vi "XNET Example IP Stack Config - Multiple VLANs.vi"(0 "XNET interface":refnum<k21>, 5 "VLANs":T1[](array[typedef]), 11 "error in (no error)":errorcluster) -> (4 "config":string, 15 "error out":errorcluster)   [LabVIEW 2018]
doc: "This example subVI generates a JSON configuration string for use with XNET IP Stack Create.vi. The configuration string supports a single XNET interface (physical interface) and one or more VLANs (virtual interfaces), each with a static IPv4 address, and a static IPv6 address.\nYou can re-use this subVI in one of two ways: a) copy the subVI from the example diagram to your VI diagram, which re-uses the subVI unchanged (located in the XNET library), or b) use Save As to create a copy of the subVI in your application folder, and change as needed."
uses:
  XNET Example IP Stack Config - Simple VLAN.ctl
  XNET Example IP Stack Config - Stack.ctl
  XNET Example IP Stack Config - XNET Interface.ctl
  XNET Example IP Stack Config - MAC.ctl
  XNET Example IP Stack Config - VLAN.ctl
  XNET Example IP Stack Config - Static Address.ctl
  XNET Example IP Stack Config - Static IPv6 Address.ctl
  XNET Example IP Stack Config - Proxy Server.ctl
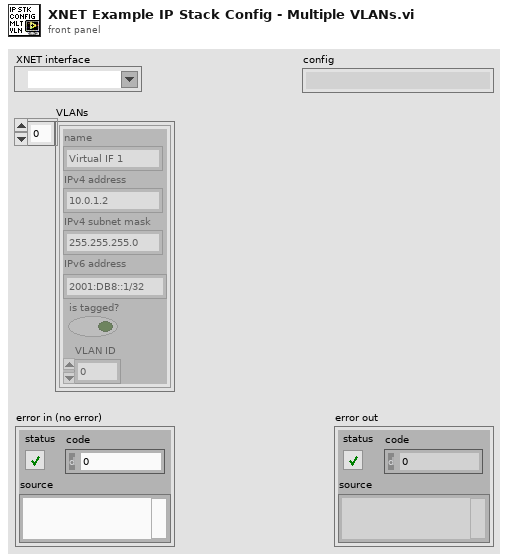
[diagram p1: front panel]
types:
  T1 = typedef "XNET Example IP Stack Config - Simple VLAN.ctl" = cluster{"name":string, "IPv4 address":string, "IPv4 subnet mask":string, "IPv6 address":string, "is tagged?":bool, "VLAN ID":u16}
  T2 = typedef "XNET Example IP Stack Config - MAC.ctl" = cluster{"address":string, "VLANs":T3[]}
  T3 = typedef "XNET Example IP Stack Config - VLAN.ctl" = cluster{"name":string, "isTagged":bool, "id":u16, "IPv4":cluster{"mode":string, "staticAddresses":T4[]}, "IPv6":cluster{"mode":string, "staticAddresses":T5[]}}
  T4 = typedef "XNET Example IP Stack Config - Static Address.ctl" = cluster{"address":string, "subnetMask":string}
  T5 = typedef "XNET Example IP Stack Config - Static IPv6 Address.ctl" = cluster{"address":string}
  T6 = typedef "XNET Example IP Stack Config - XNET Interface.ctl" = cluster{"name":string, "MACs":T2[]}
  T7 = typedef "XNET Example IP Stack Config - Stack.ctl" = cluster{"schema":string, "xnetInterfaces":T6[], "proxyServers":T8[]}
  T8 = typedef "XNET Example IP Stack Config - Proxy Server.ctl" = cluster{"protocol":string, "direction":string, "listenAddress":string, "listenPort":u16, "forwardingDestinationAddress":string, "forwardingDestinationPort":u16, "forwardingSourceAddress":string, "forwardingSourcePort":u16}
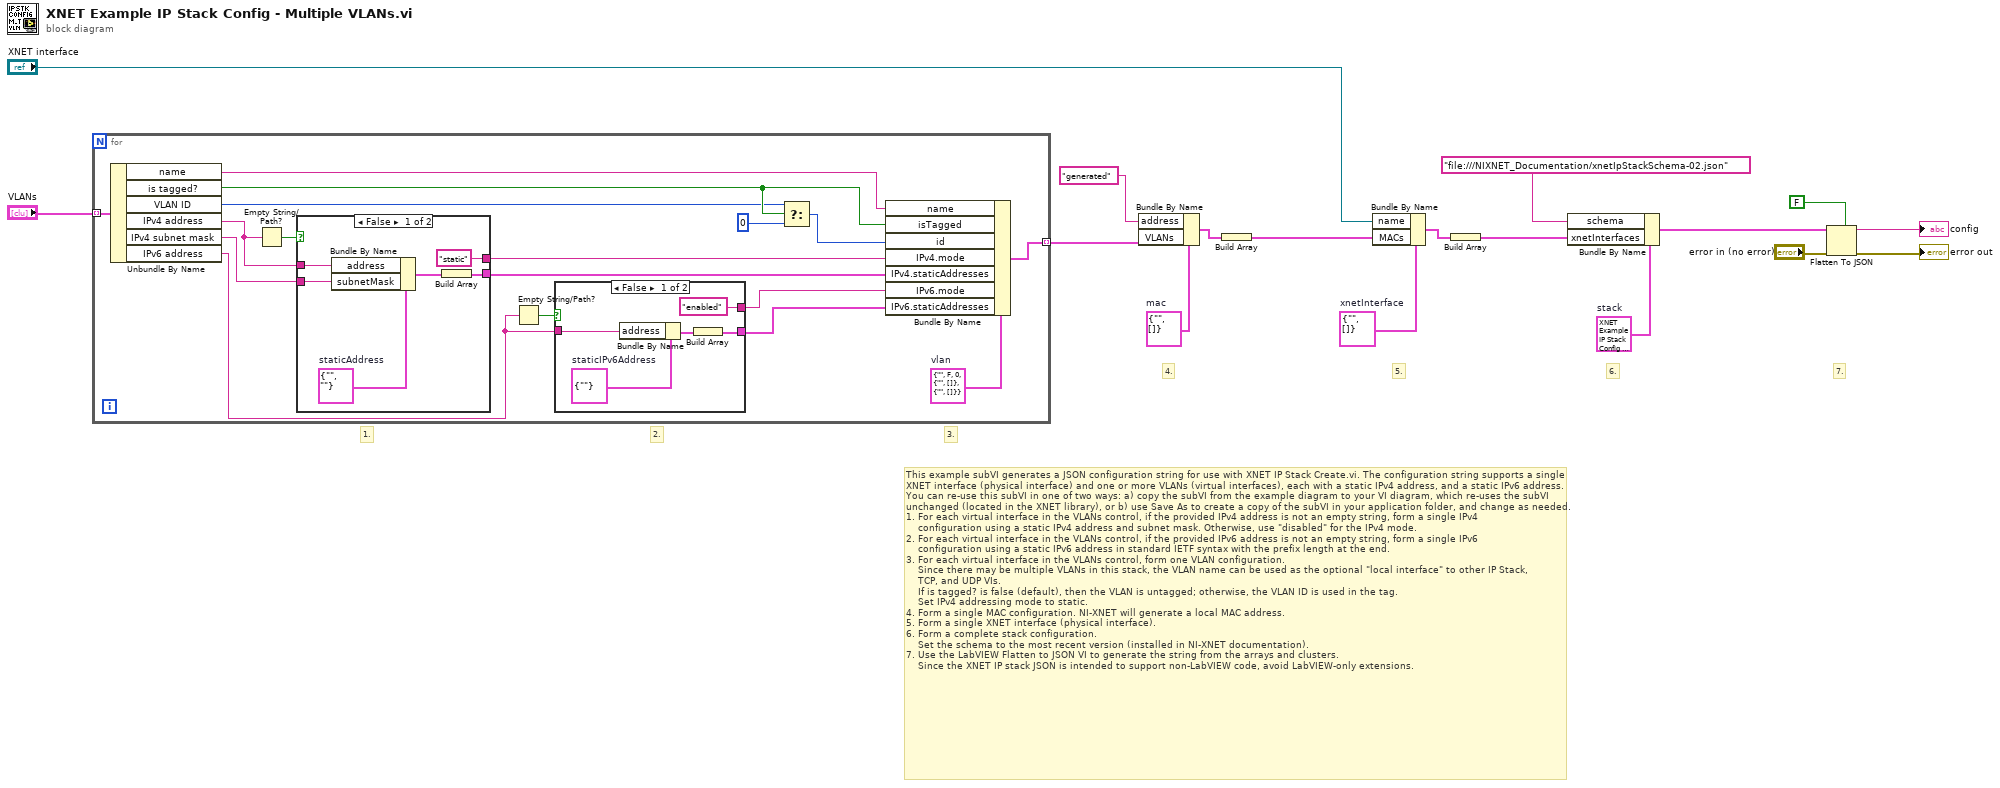
[diagram p0: block diagram]
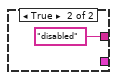
[diagram p2: hidden frame]
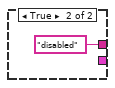
[diagram p3: hidden frame]
diagram:
  w6 = T2 {"address"="", "VLANs"=[]}  # mac
  w9 = T6 {"name"="", "MACs"=[]}  # xnetInterface
  w10 = T7 {"schema"="", "xnetInterfaces"=[{"name"="", "MACs"=[{"address"="", "VLANs"=[{"name"="", "isTagged"=FALSE, "id"=0, "IPv4"={"mode"="static", "staticAddresses"=[]}, "IPv6"={"mode"="", "staticAddresses"=[]}}]}]}], "proxyServers"=[]}  # stack
  # "2."
  # "1."
  # "3."
  # "7."
  # "6."
  # "5."
  # "4."
  # "This example subVI generates a JSON configuration string for use with XNET IP Stack Create.vi. The configuration string supports a single XNET interface (physical interface) and one or more VLANs (virtual interfaces), each with a static IPv4 address, and a static IPv6 address.\nYou can re-use this subVI in one of two ways: a) copy the subVI from the example diagram to your VI diagram, which re-uses the subVI unchanged (located in the XNET library), or b) use Save As to create a copy of the subVI in your application folder, and change as needed.\n1. For each virtual interface in the VLANs control, if the provided IPv4 address is not an empty string, form a single IPv4\n    configuration using a static IPv4 address and subnet mask. Otherwise, use \"disabled\" for the IPv4 mode.\n2. For each virtual interface in the VLANs control, if the provided IPv6 address is not an empty string, form a single IPv6\n    configuration using a static IPv6 address in standard IETF syntax with the prefix length at the end.\n3. For each virtual interface in the VLANs control, form one VLAN configuration.\n    Since there may be multiple VLANs in this stack, the VLAN name can be used as the optional \"local interface\" to other IP Stack,     \n    TCP, and UDP VIs.\n    If is tagged? is false (default), then the VLAN is untagged; otherwise, the VLAN ID is used in the tag.\n    Set IPv4 addressing mode to static.\n4. Form a single MAC configuration. NI-XNET will generate a local MAC address.\n5. Form a single XNET interface (physical interface).\n6. Form a complete stack configuration.\n    Set the schema to the most recent version (installed in NI-XNET documentation).\n7. Use the LabVIEW Flatten to JSON VI to generate the string from the arrays and clusters.\n    Since the XNET IP stack JSON is intended to support non-LabVIEW code, avoid LabVIEW-only extensions."
  n1 = for {
    tunnel: [w31] -> w2 mode=indexing
    tunnel: "VLANs" -> [w30] mode=indexing
    w34 = T3 {"name"="", "isTagged"=FALSE, "id"=0, "IPv4"={"mode"="", "staticAddresses"=[]}, "IPv6"={"mode"="", "staticAddresses"=[]}}  # vlan
    n2 = Unbundle By Name(w30) -> ("name"=w29:string, "is tagged?"=w28:bool, "VLAN ID"=w18:u16, "IPv4 address"=w25:string, "IPv4 subnet mask"=w24:string, "IPv6 address"=w23:string)
    n3 = Empty String/Path?(string/path=w25) -> (empty?=w27:bool)
    n4 = case shown="False" w27 {
      tunnel: [w44 _] -> w21
      tunnel: w24 -> [w43 _]
      tunnel: w25 -> [w42 _]
      tunnel: ["static" ("IPv4.mode") "disabled" ("IPv4.mode")] -> w22
      frame False {
        w45 = T4 {"address"="", "subnetMask"=""}  # staticAddress
        n5 = Bundle By Name(cluster=w45, "address"=w42, "subnetMask"=w43) -> (w46:T4)
        n6 = Build Array(w46) -> (w44:T4[])
      }
      frame True {
      }
    }
    n7 = Empty String/Path?(string/path=w23) -> (empty?=w26:bool)
    n8 = case shown="False" w26 {
      tunnel: w23 -> [w35 _]
      tunnel: [w39 _] -> w19
      tunnel: ["enabled" ("IPv4.mode") "disabled" ("IPv4.mode")] -> w20
      frame False {
        w37 = T5 {"address"=""}  # staticIPv6Address
        n9 = Bundle By Name(cluster=w37, "address"=w35) -> (w36:T5)
        n10 = Build Array(w36) -> (w39:T5[])
      }
      frame True {
      }
    }
    n11 = Select(t=w18, s=w28, f=u16 0) -> (s? t:f=w32:u16)
    n12 = Bundle By Name(cluster=w34, "name"=w29, "isTagged"=w28, "id"=w32, "IPv4.mode"=w22, "IPv4.staticAddresses"=w21, "IPv6.mode"=w20, "IPv6.staticAddresses"=w19) -> (w31:T3)
  }
  n13 = Bundle By Name(cluster=w6, "address"="generated", "VLANs"=w2) -> (w7:T2)
  n14 = Build Array(w7) -> (w5:T2[])
  n15 = Bundle By Name(cluster=w9, "name"="XNET interface", "MACs"=w5) -> (w8:T6)
  n16 = Build Array(w8) -> (w11:T6[])
  n17 = Bundle By Name(cluster=w10, "schema"="file:///NIXNET_Documentation/xnetIpStackSchema-02.json", "xnetInterfaces"=w11) -> (w13:T7)
  n18 = Flatten To JSON(enable LabVIEW extensions? (T)=FALSE, anything=w13, error in (no error)="error in (no error)") -> (JSON string=→"config":string, 11:→"error out":errorcluster)
